vi "RQ - Generate service request (SRQ).vi"(1 "Generate interrupt and set\nbits: nn":dbl format="%.2f", 2 "error in":errorcluster, 3 "Address / Port":i16=1 min=1 max=31 step=1) -> (0 "error out":errorcluster)   [LabVIEW 2014]
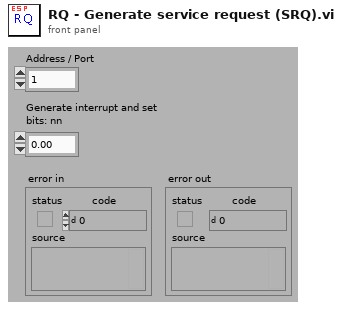
[diagram p1: front panel]
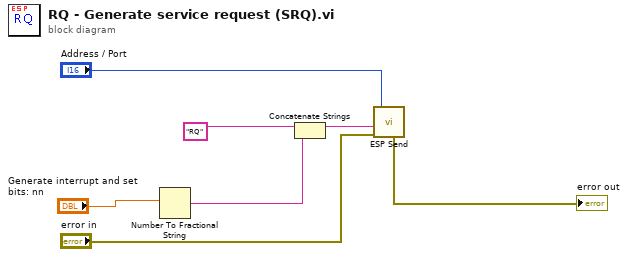
[diagram p0: block diagram]
diagram:
  n1 = Number To Fractional String(number="Generate interrupt and set\nbits: nn") -> (F-format string=w1:string)  [unwired: 3 in]
  n2 = Concatenate Strings("RQ" ("Substring"), w1) -> (w6:string)
  n3 = call "ESP Send.vi"("Address / Port"="Address / Port", "Command String"=w6, "error in"="error in") -> ("error out"=→"error out":errorcluster)  [unwired: 5 in]
